vi "VSG25_Main.vi"() -> ()   [LabVIEW 2014]
uses:
  Queue Control.ctl
  sg_lib/VSG25A.lvlib
panel:
  in  "Arb Button":bool
  in  "CW Button":bool
  in  "StepSweep Button":bool
  in  "RampSweep Button":bool
  in  "QAM Button":bool
  in  "FSK Button":bool
  in  "Multitone Button":bool
  in  "Pulse Button":bool
  in  "FM Button":bool
  in  "AM Button":bool
  in  "Exit Button":bool caption="Blank Button"
  in  "Error In":errorcluster
  in  "Connect Button":bool caption="Blank Button"
  out "Error Out":errorcluster
  # "Vector Signal Generator"
  # "Signal Hound VSG25"
  # "Operational Modes:"
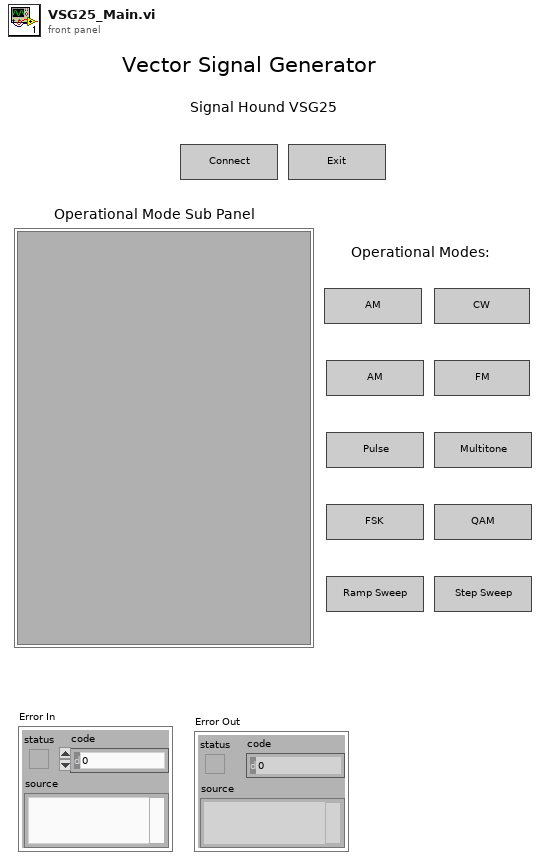
[diagram p1: front panel]
types:
  T1 = typedef "Queue Control.ctl" = cluster{"Command":enum16{"Pulse", "AM", "FM", "Connect", "Exit", "RF On", "CW", "StepSweep", "RampSweep"}, "Data":variant}
  T2 = enum16{"Init", "Proc GUI Events", "Dispatch", "Exit"}
  T3 = enum16{"Pulse", "AM", "FM", "Connect", "Exit", "RF On", "CW", "StepSweep", "RampSweep"}
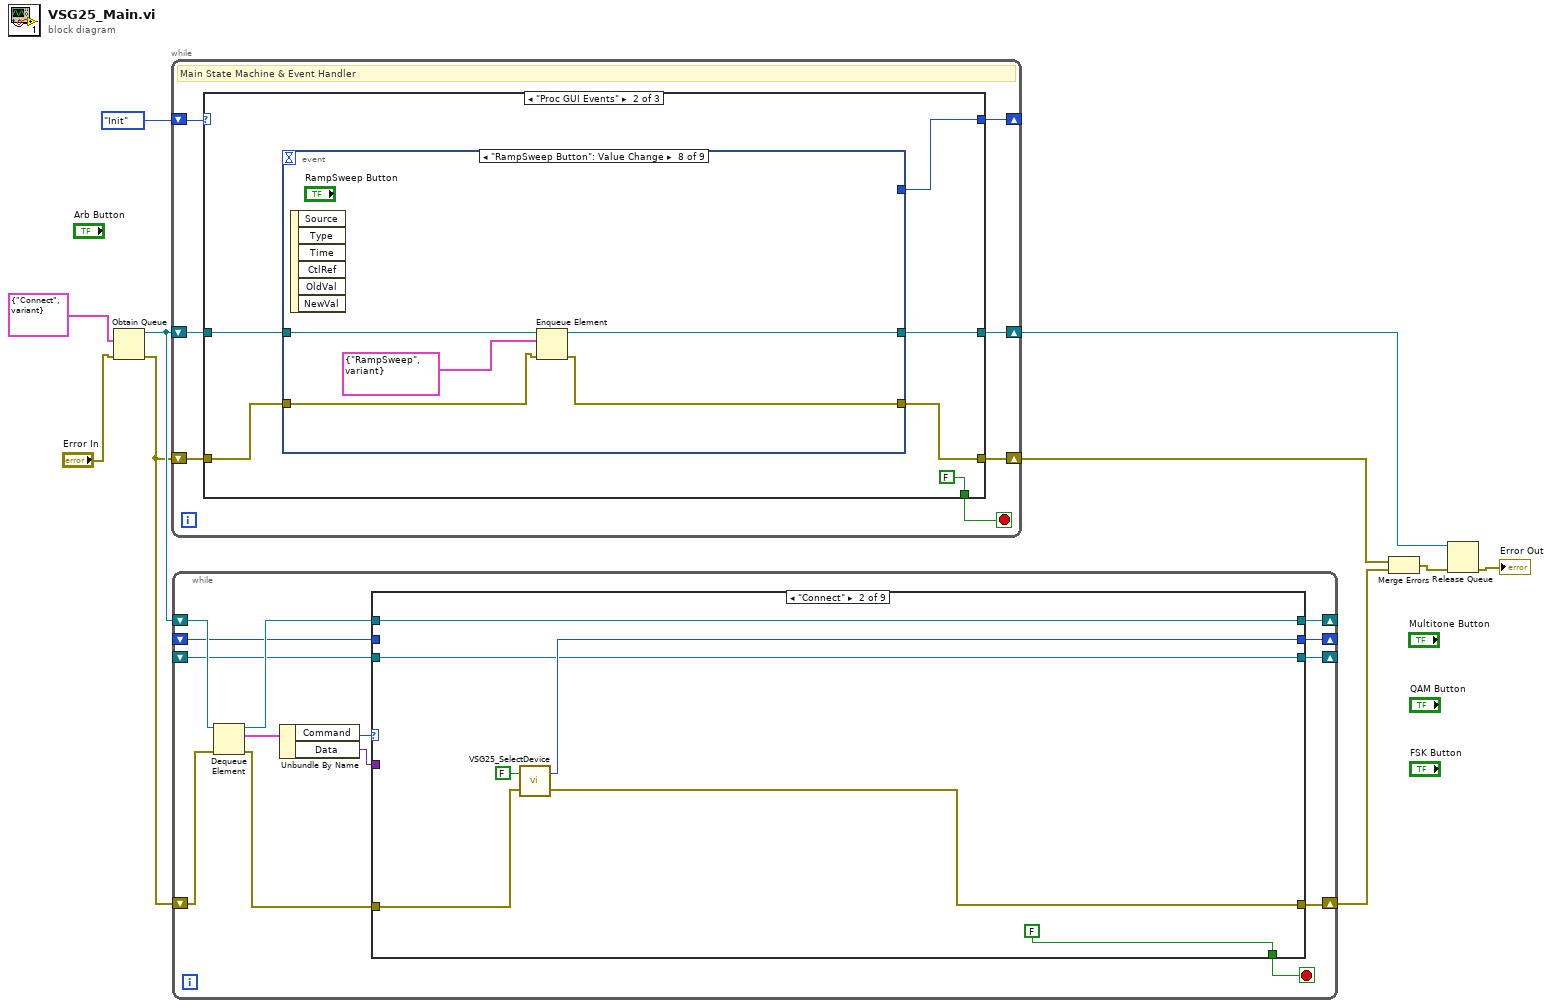
[diagram p0: block diagram]
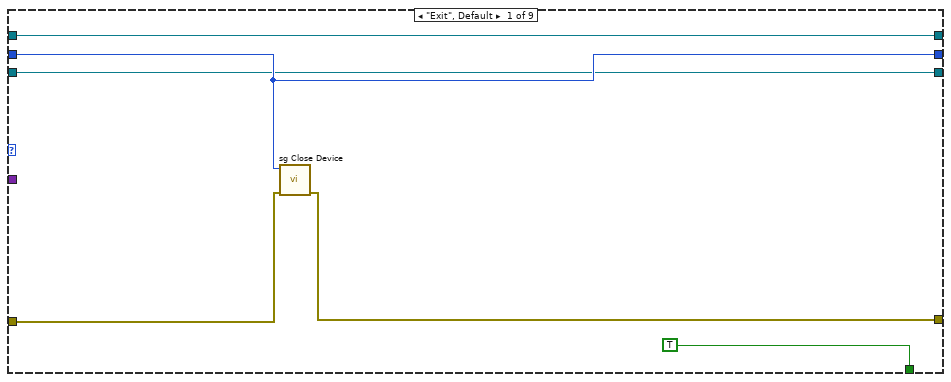
[diagram p2: hidden frame]
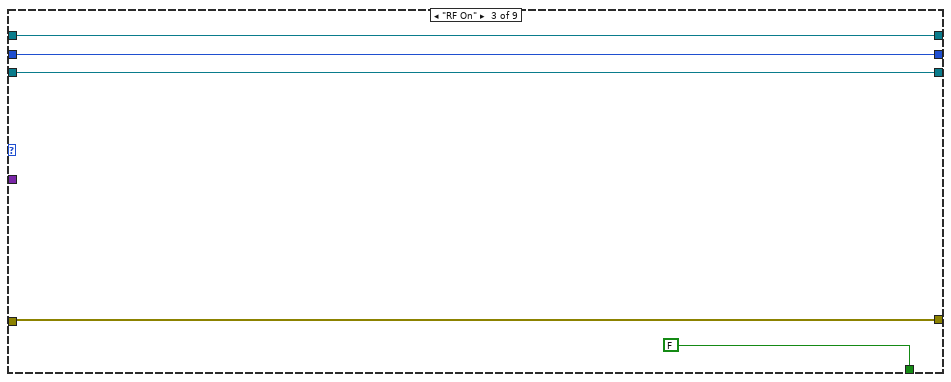
[diagram p3: hidden frame]
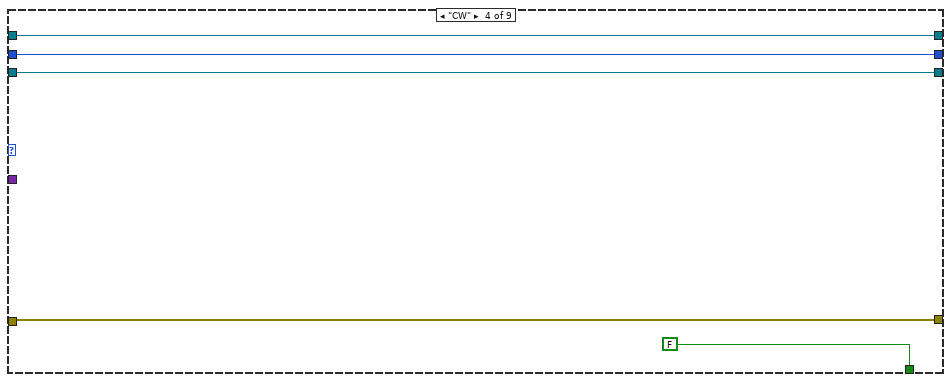
[diagram p4: hidden frame]
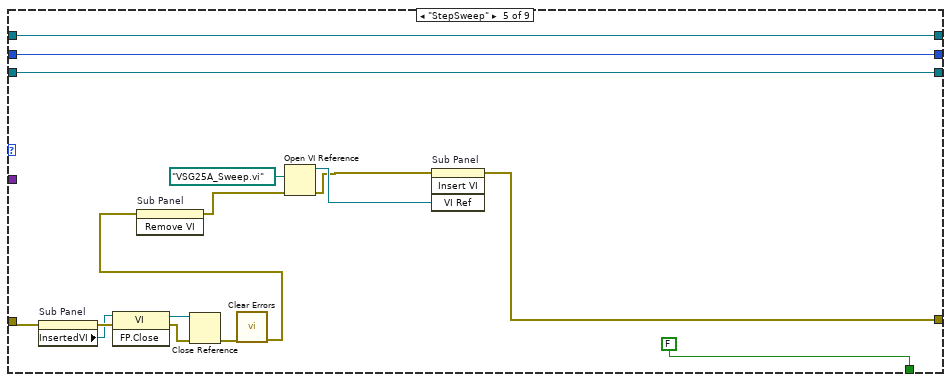
[diagram p5: hidden frame]
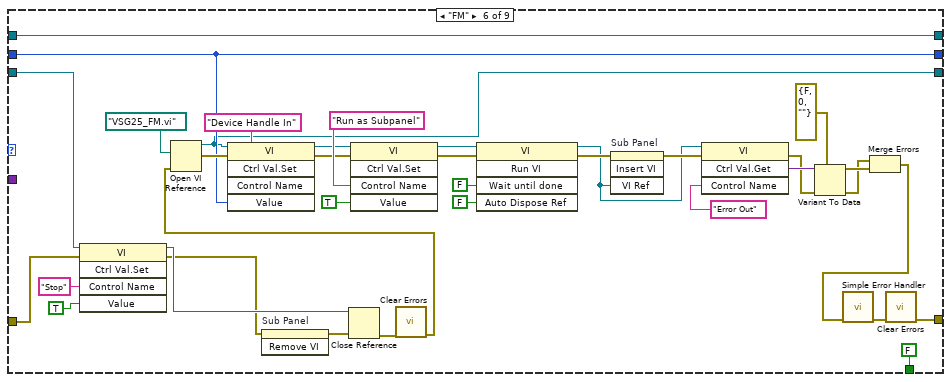
[diagram p6: hidden frame]
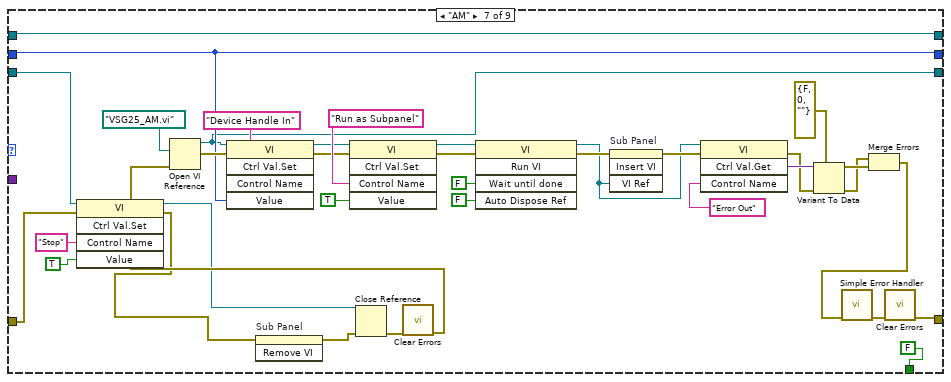
[diagram p7: hidden frame]
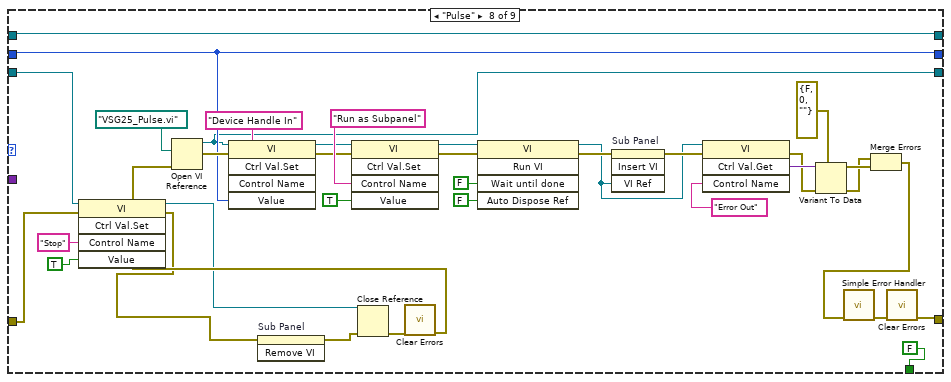
[diagram p8: hidden frame]
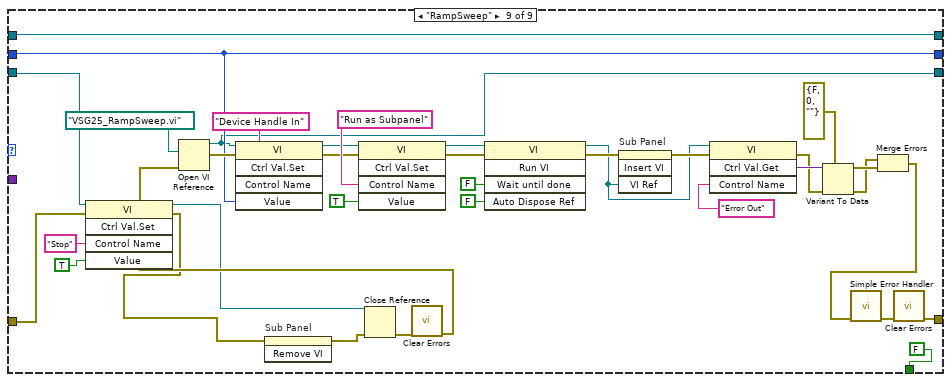
[diagram p9: hidden frame]
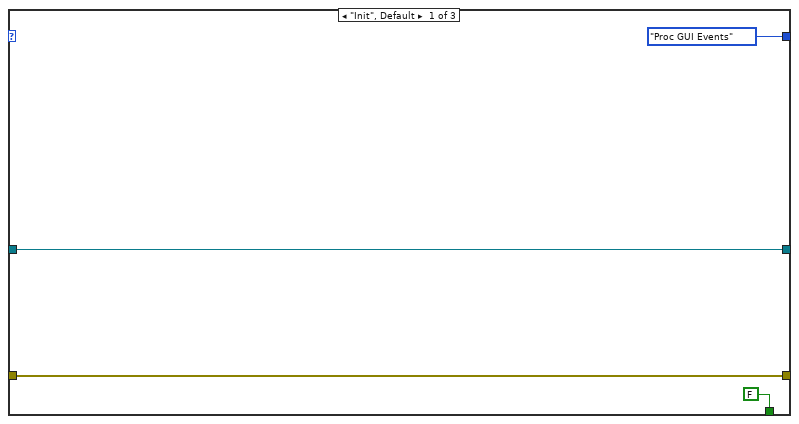
[diagram p10: hidden frame]
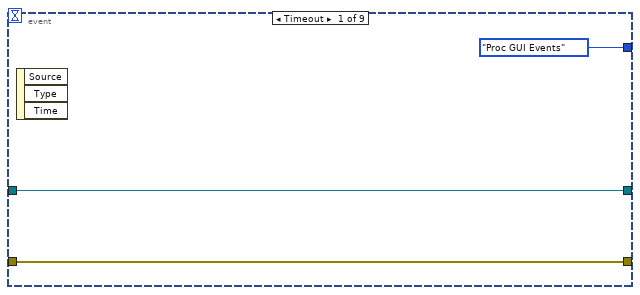
[diagram p11: hidden frame]
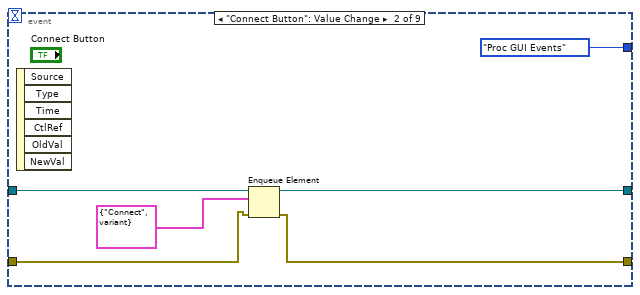
[diagram p12: hidden frame]
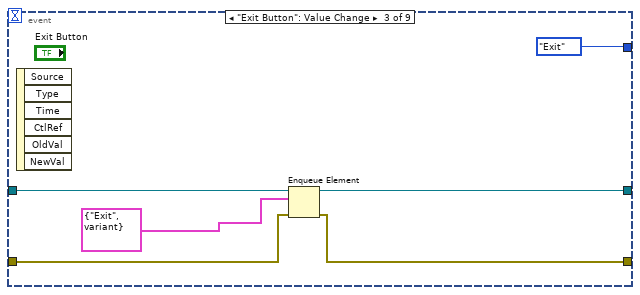
[diagram p13: hidden frame]
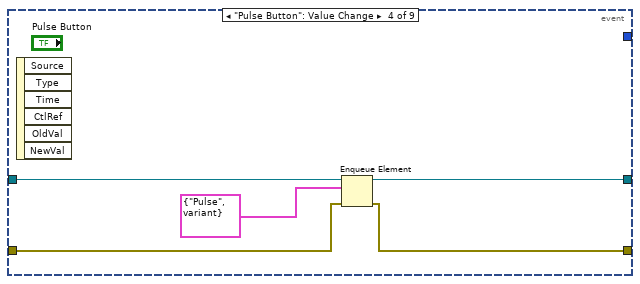
[diagram p14: hidden frame]
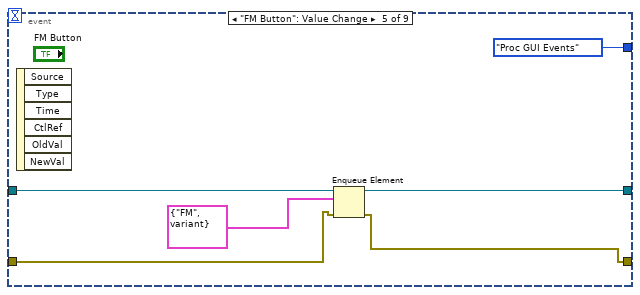
[diagram p15: hidden frame]
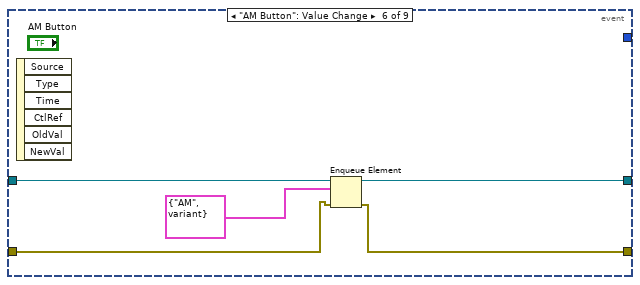
[diagram p16: hidden frame]
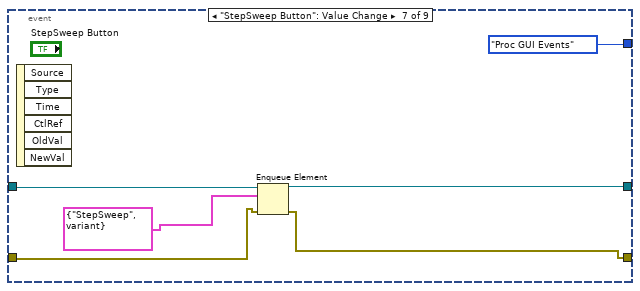
[diagram p17: hidden frame]
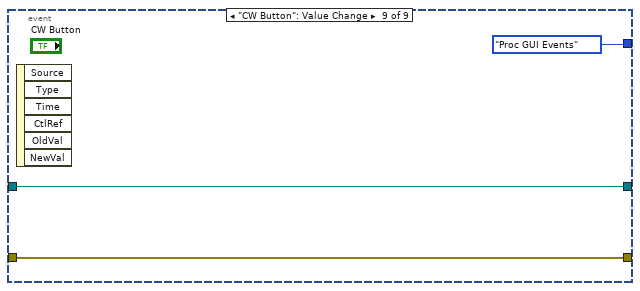
[diagram p18: hidden frame]
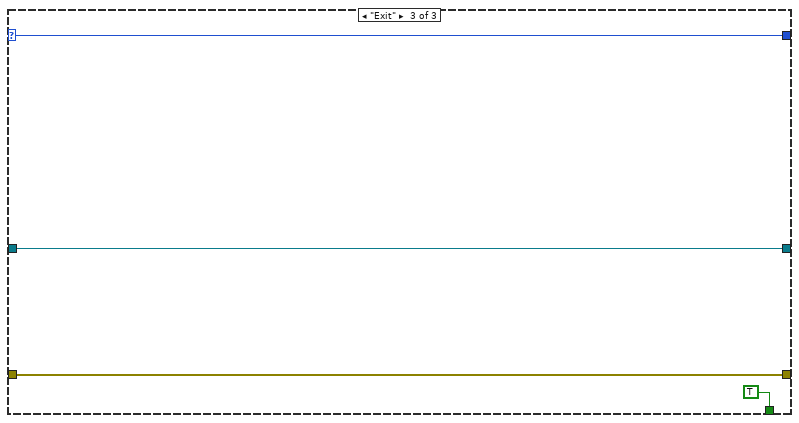
[diagram p19: hidden frame]
diagram:
  n1 = Obtain Queue(element data type=T1 {"Command"=enum."Connect", "Data"=variant} ("Queue Cluster"), error in (no error)="Error In") -> (queue out=w7:refnum<queue>, error out=w1:errorcluster)  [unwired: 3 in, 1 out]
  n2 = while {
    shift-right: [w14] -> _
    shift-left: T2."Init" -> [w17]
    shift-right: [w12] -> w3
    shift-left: w7 -> [w13]
    shift-right: [w11] -> w5
    shift-left: w1 -> [w16]
    stop <- w15 stop-if-true
    # "Main State Machine & Event Handler"
    n3 = case shown="\"Proc GUI Events\"" w17 {
      selector: w17 -> [_ _ w75]
      tunnel: w16 -> [w18 w23 w73]
      tunnel: [FALSE FALSE TRUE] -> w15
      tunnel: [T2."Proc GUI Events" w26 w75] -> w14
      tunnel: w13 -> [w19 w25 w74]
      tunnel: [w19 w24 w74] -> w12
      tunnel: [w18 w22 w73] -> w11
      frame "Init", Default {
      }
      frame "Proc GUI Events" {
        n4 = event shown="[7] \"RampSweep Button\": Value Change" {
          selector: _ -> [_ _ _ _ _ _ _ _ _]
          dyn-events: _ -> [_ _ _ _ _ _ _ _ _]
          timeout: _ -> [_ _ _ _ _ _ _ _ _]
          tunnel: [T2."Proc GUI Events" T2."Proc GUI Events" T2."Exit" _ T2."Proc GUI Events" _ T2."Proc GUI Events" _ T2."Proc GUI Events"] -> w26
          tunnel: w25 -> [w29 w35 w41 w46 w49 w56 w64 w68 w72]
          tunnel: [w29 w34 w40 w43 w50 w57 w61 w65 w72] -> w24
          tunnel: w23 -> [w28 w33 w39 w45 w48 w55 w63 w67 w71]
          tunnel: [w28 w32 w38 w44 w51 w54 w62 w66 w71] -> w22
          event Timeout {
            n5 = event-data() -> ()  [unwired: 1 in, 3 out]
          }
          event "Connect Button": Value Change {
            n6 = event-data() -> ()  [unwired: 1 in, 6 out]
            n7 = Enqueue Element(queue=w35, element=T1 {"Command"=enum."Connect", "Data"=variant} ("Queue Cluster"), error in (no error)=w33) -> (queue out=w34:refnum<queue>, error out=w32:errorcluster)  [unwired: 1 in, 1 out]
          }
          event "Exit Button": Value Change {
            n8 = event-data() -> ()  [unwired: 1 in, 6 out]
            n9 = Enqueue Element(queue=w41, element=T1 {"Command"=enum."Exit", "Data"=variant} ("Queue Cluster"), error in (no error)=w39) -> (queue out=w40:refnum<queue>, error out=w38:errorcluster)  [unwired: 1 in, 1 out]
          }
          event "Pulse Button": Value Change {
            n10 = event-data() -> ()  [unwired: 1 in, 6 out]
            n11 = Enqueue Element(queue=w46, element=T1 {"Command"=enum."Pulse", "Data"=variant} ("Queue Cluster"), error in (no error)=w45) -> (queue out=w43:refnum<queue>, error out=w44:errorcluster)  [unwired: 1 in, 1 out]
          }
          event "FM Button": Value Change {
            n12 = event-data() -> ()  [unwired: 1 in, 6 out]
            n13 = Enqueue Element(queue=w49, element=T1 {"Command"=enum."FM", "Data"=variant} ("Queue Cluster"), error in (no error)=w48) -> (queue out=w50:refnum<queue>, error out=w51:errorcluster)  [unwired: 1 in, 1 out]
          }
          event "AM Button": Value Change {
            n14 = event-data() -> ()  [unwired: 1 in, 6 out]
            n15 = Enqueue Element(queue=w56, element=T1 {"Command"=enum."AM", "Data"=variant} ("Queue Cluster"), error in (no error)=w55) -> (queue out=w57:refnum<queue>, error out=w54:errorcluster)  [unwired: 1 in, 1 out]
          }
          event "StepSweep Button": Value Change {
            n16 = event-data() -> ()  [unwired: 1 in, 6 out]
            n17 = Enqueue Element(queue=w64, element=T1 {"Command"=enum."StepSweep", "Data"=variant} ("Queue Cluster"), error in (no error)=w63) -> (queue out=w61:refnum<queue>, error out=w62:errorcluster)  [unwired: 1 in, 1 out]
          }
          event "RampSweep Button": Value Change {
            n18 = event-data() -> ()  [unwired: 1 in, 6 out]
            n19 = Enqueue Element(queue=w68, element=T1 {"Command"=enum."RampSweep", "Data"=variant} ("Queue Cluster"), error in (no error)=w67) -> (queue out=w65:refnum<queue>, error out=w66:errorcluster)  [unwired: 1 in, 1 out]
          }
          event "CW Button": Value Change {
            n20 = event-data() -> ()  [unwired: 1 in, 6 out]
          }
        }
      }
      frame "Exit" {
      }
    }
  }
  n21 = while {
    shift-right: [w88] -> _
    shift-left: w7 -> [w90]
    shift-right: [w86] -> w6
    shift-left: w1 -> [w85]
    shift-right: [w82] -> _
    shift-left: _ -> [w81]
    shift-right: [w78] -> _
    shift-left: _ -> [w77]
    stop <- w80 stop-if-true
    n22 = Dequeue Element(queue=w90, error in (no error)=w85) -> (queue out=w89:refnum<queue>, element=w84:T1, error out=w87:errorcluster)  [unwired: 1 in, 1 out]
    n23 = Unbundle By Name(w84) -> ("Command"=w83:T3, "Data"=w79:variant)
    n24 = case shown="\"Connect\"" w83 {
      tunnel: w89 -> [w93 w103 w106 w111 w124 w164 w177 w205 w243]
      tunnel: [w93 w103 w106 w111 w124 w164 w177 w205 w243] -> w88
      tunnel: w87 -> [w95 w102 w105 w110 w116 w130 w166 w207 w240]
      tunnel: [w94 w98 w105 w110 w122 w139 w175 w202 w239] -> w86
      tunnel: [w96 w101 w107 w112 w125 w156 w178 w204 w242] -> w82
      tunnel: w81 -> [w96 _ w107 w112 w125 w156 w178 w204 w242]
      tunnel: [TRUE ("AutoSel") FALSE ("AutoSel") FALSE ("AutoSel") FALSE ("AutoSel") FALSE ("AutoSel") FALSE ("AutoSel") FALSE ("AutoSel") FALSE ("AutoSel") FALSE ("AutoSel")] -> w80
      tunnel: w79 -> [_ _ _ _ _ _ _ _ _]
      tunnel: [w91 w97 w104 w109 w114 w137 w173 w203 w241] -> w78
      tunnel: w77 -> [w91 w97 w104 w109 w114 w131 w170 w206 w244]
      frame "Exit", Default {
        n25 = call "sg Close Device.vi"("error in (no error)"=w95, "device"=w96) -> ("error out"=w94:errorcluster)  [unwired: 8 in, 1 out]
      }
      frame "Connect" {
        n26 = call "VSG25_SelectDevice.vi"("ErrorIn"=w102, "AutoSel"=FALSE) -> ("ErrorOut"=w98:errorcluster, "deviceHandle"=w101:i32)
      }
      frame "RF On" {
      }
      frame "CW" {
      }
      frame "StepSweep" {
        n27 = property on="Sub Panel" class="SubPnl"(error in=w116) -> (error out=w119:errorcluster, "InsertedVI"=w118:refnum<vi>)  [unwired: 1 in, 1 out]
        n28 = invoke class="VI" method="FP.Close"(reference=w118, error in=w119) -> (reference out=w121:refnum<vi>, error out=w120:errorcluster)  [unwired: 1 in, 1 out]
        n29 = Close Reference(reference=w121, error in (no error)=w120) -> (error out=w117:errorcluster)
        n30 = call <vilib>:"Clear Errors.vi"("error in (no error)"=w117) -> ("error out"=w115:errorcluster)  [unwired: 5 in, 1 out]
        n31 = invoke on="Sub Panel" class="SubPnl" method="Remove VI"(error in=w115) -> (error out=w123:errorcluster)  [unwired: 2 in, 2 out]
        n32 = Open VI Reference(vi path=path "VSG25A_Sweep.vi", error in (no error)=w123) -> (vi reference=w128:refnum<vi>, error out=w127:errorcluster)  [unwired: 4 in]
        n33 = invoke on="Sub Panel" class="SubPanel" method="Insert VI"(error in=w127, "VI Ref"=w128) -> (error out=w122:errorcluster)  [unwired: 2 in, 3 out]
      }
      frame "FM" {
        n34 = invoke class="VI" method="Ctrl Val.Set"(reference=w131, error in=w130, "Control Name"="Stop", "Value"=TRUE) -> (reference out=w133:refnum<vi>, error out=w132:errorcluster)  [unwired: 1 in, 3 out]
        n35 = invoke on="Sub Panel" class="SubPnl" method="Remove VI"(error in=w132) -> (error out=w136:errorcluster)  [unwired: 2 in, 2 out]
        n36 = Close Reference(reference=w133, error in (no error)=w136) -> (error out=w142:errorcluster)
        n37 = call <vilib>:"Clear Errors.vi"("error in (no error)"=w142) -> ("error out"=w138:errorcluster)  [unwired: 5 in, 1 out]
        n38 = Open VI Reference(vi path=path "VSG25_FM.vi", error in (no error)=w138) -> (vi reference=w137:refnum<vi>, error out=w159:errorcluster)  [unwired: 4 in]
        n39 = invoke class="VI" method="Ctrl Val.Set"(reference=w137, error in=w159, "Control Name"="Device Handle In", "Value"=w156) -> (reference out=w157:refnum<vi>, error out=w158:errorcluster)  [unwired: 1 in, 3 out]
        n40 = invoke class="VI" method="Ctrl Val.Set"(reference=w157, error in=w158, "Control Name"="Run as Subpanel", "Value"=TRUE) -> (reference out=w155:refnum<vi>, error out=w152:errorcluster)  [unwired: 1 in, 3 out]
        n41 = invoke class="VI" method="Run VI"(reference=w155, error in=w152, "Wait until done"=FALSE ("Wait Until Done"), "Auto Dispose Ref"=FALSE ("Auto Dispose Reference")) -> (reference out=w148:refnum<vi>, error out=w151:errorcluster)  [unwired: 1 in, 3 out]
        n42 = invoke on="Sub Panel" class="SubPanel" method="Insert VI"(error in=w151, "VI Ref"=w148) -> (error out=w149:errorcluster)  [unwired: 2 in, 3 out]
        n43 = invoke class="VI" method="Ctrl Val.Get"(reference=w148, error in=w149, "Control Name"="Error Out") -> (error out=w144:errorcluster, "Get Control Value Variant"=w147:variant)  [unwired: 1 in, 2 out]
        n44 = Variant To Data(error in=w144, type=errorcluster {"status"=FALSE, "code"=0, "source"=""} ("error constant"), Variant=w147) -> (data=w145:errorcluster, error out=w143:errorcluster)
        n45 = Merge Errors(w143, w145) -> (w141:errorcluster)
        n46 = call <vilib>:"Simple Error Handler.vi"("error in (no error)"=w141) -> ("error out"=w140:errorcluster)  [unwired: 4 in, 4 out]
        n47 = call <vilib>:"Clear Errors.vi"("error in (no error)"=w140) -> ("error out"=w139:errorcluster)  [unwired: 5 in, 1 out]
      }
      frame "AM" {
        n48 = invoke class="VI" method="Ctrl Val.Set"(reference=w170, error in=w166, "Control Name"="Stop", "Value"=TRUE) -> (reference out=w168:refnum<vi>, error out=w167:errorcluster)  [unwired: 1 in, 3 out]
        n49 = invoke on="Sub Panel" class="SubPnl" method="Remove VI"(error in=w167) -> (error out=w169:errorcluster)  [unwired: 2 in, 2 out]
        n50 = Close Reference(reference=w168, error in (no error)=w169) -> (error out=w181:errorcluster)
        n51 = call <vilib>:"Clear Errors.vi"("error in (no error)"=w181) -> ("error out"=w174:errorcluster)  [unwired: 5 in, 1 out]
        n52 = Open VI Reference(vi path=path "VSG25_AM.vi", error in (no error)=w174) -> (vi reference=w173:refnum<vi>, error out=w197:errorcluster)  [unwired: 4 in]
        n53 = invoke class="VI" method="Ctrl Val.Set"(reference=w173, error in=w197, "Control Name"="Device Handle In", "Value"=w178) -> (reference out=w195:refnum<vi>, error out=w196:errorcluster)  [unwired: 1 in, 3 out]
        n54 = invoke class="VI" method="Ctrl Val.Set"(reference=w195, error in=w196, "Control Name"="Run as Subpanel", "Value"=TRUE) -> (reference out=w194:refnum<vi>, error out=w191:errorcluster)  [unwired: 1 in, 3 out]
        n55 = invoke class="VI" method="Run VI"(reference=w194, error in=w191, "Wait until done"=FALSE ("Wait Until Done"), "Auto Dispose Ref"=FALSE ("Auto Dispose Reference")) -> (reference out=w187:refnum<vi>, error out=w190:errorcluster)  [unwired: 1 in, 3 out]
        n56 = invoke on="Sub Panel" class="SubPanel" method="Insert VI"(error in=w190, "VI Ref"=w187) -> (error out=w188:errorcluster)  [unwired: 2 in, 3 out]
        n57 = invoke class="VI" method="Ctrl Val.Get"(reference=w187, error in=w188, "Control Name"="Error Out") -> (error out=w183:errorcluster, "Get Control Value Variant"=w186:variant)  [unwired: 1 in, 2 out]
        n58 = Variant To Data(error in=w183, type=errorcluster {"status"=FALSE, "code"=0, "source"=""} ("error constant"), Variant=w186) -> (data=w184:errorcluster, error out=w182:errorcluster)
        n59 = Merge Errors(w182, w184) -> (w180:errorcluster)
        n60 = call <vilib>:"Simple Error Handler.vi"("error in (no error)"=w180) -> ("error out"=w179:errorcluster)  [unwired: 4 in, 4 out]
        n61 = call <vilib>:"Clear Errors.vi"("error in (no error)"=w179) -> ("error out"=w175:errorcluster)  [unwired: 5 in, 1 out]
      }
      frame "Pulse" {
        n62 = invoke class="VI" method="Ctrl Val.Set"(reference=w206, error in=w207, "Control Name"="Stop", "Value"=TRUE) -> (reference out=w210:refnum<vi>, error out=w209:errorcluster)  [unwired: 1 in, 3 out]
        n63 = invoke on="Sub Panel" class="SubPnl" method="Remove VI"(error in=w209) -> (error out=w211:errorcluster)  [unwired: 2 in, 2 out]
        n64 = Close Reference(reference=w210, error in (no error)=w211) -> (error out=w217:errorcluster)
        n65 = call <vilib>:"Clear Errors.vi"("error in (no error)"=w217) -> ("error out"=w214:errorcluster)  [unwired: 5 in, 1 out]
        n66 = Open VI Reference(vi path=path "VSG25_Pulse.vi", error in (no error)=w214) -> (vi reference=w203:refnum<vi>, error out=w233:errorcluster)  [unwired: 4 in]
        n67 = invoke class="VI" method="Ctrl Val.Set"(reference=w203, error in=w233, "Control Name"="Device Handle In", "Value"=w204) -> (reference out=w231:refnum<vi>, error out=w232:errorcluster)  [unwired: 1 in, 3 out]
        n68 = invoke class="VI" method="Ctrl Val.Set"(reference=w231, error in=w232, "Control Name"="Run as Subpanel", "Value"=TRUE) -> (reference out=w230:refnum<vi>, error out=w227:errorcluster)  [unwired: 1 in, 3 out]
        n69 = invoke class="VI" method="Run VI"(reference=w230, error in=w227, "Wait until done"=FALSE ("Wait Until Done"), "Auto Dispose Ref"=FALSE ("Auto Dispose Reference")) -> (reference out=w223:refnum<vi>, error out=w226:errorcluster)  [unwired: 1 in, 3 out]
        n70 = invoke on="Sub Panel" class="SubPanel" method="Insert VI"(error in=w226, "VI Ref"=w223) -> (error out=w224:errorcluster)  [unwired: 2 in, 3 out]
        n71 = invoke class="VI" method="Ctrl Val.Get"(reference=w223, error in=w224, "Control Name"="Error Out") -> (error out=w219:errorcluster, "Get Control Value Variant"=w222:variant)  [unwired: 1 in, 2 out]
        n72 = Variant To Data(error in=w219, type=errorcluster {"status"=FALSE, "code"=0, "source"=""} ("error constant"), Variant=w222) -> (data=w220:errorcluster, error out=w218:errorcluster)
        n73 = Merge Errors(w218, w220) -> (w216:errorcluster)
        n74 = call <vilib>:"Simple Error Handler.vi"("error in (no error)"=w216) -> ("error out"=w215:errorcluster)  [unwired: 4 in, 4 out]
        n75 = call <vilib>:"Clear Errors.vi"("error in (no error)"=w215) -> ("error out"=w202:errorcluster)  [unwired: 5 in, 1 out]
      }
      frame "RampSweep" {
        n76 = invoke class="VI" method="Ctrl Val.Set"(reference=w244, error in=w240, "Control Name"="Stop", "Value"=TRUE) -> (reference out=w246:refnum<vi>, error out=w245:errorcluster)  [unwired: 1 in, 3 out]
        n77 = invoke on="Sub Panel" class="SubPnl" method="Remove VI"(error in=w245) -> (error out=w247:errorcluster)  [unwired: 2 in, 2 out]
        n78 = Close Reference(reference=w246, error in (no error)=w247) -> (error out=w253:errorcluster)
        n79 = call <vilib>:"Clear Errors.vi"("error in (no error)"=w253) -> ("error out"=w250:errorcluster)  [unwired: 5 in, 1 out]
        n80 = Open VI Reference(vi path=path "VSG25_RampSweep.vi", error in (no error)=w250) -> (vi reference=w241:refnum<vi>, error out=w269:errorcluster)  [unwired: 4 in]
        n81 = invoke class="VI" method="Ctrl Val.Set"(reference=w241, error in=w269, "Control Name"="Device Handle In", "Value"=w242) -> (reference out=w267:refnum<vi>, error out=w268:errorcluster)  [unwired: 1 in, 3 out]
        n82 = invoke class="VI" method="Ctrl Val.Set"(reference=w267, error in=w268, "Control Name"="Run as Subpanel", "Value"=TRUE) -> (reference out=w266:refnum<vi>, error out=w263:errorcluster)  [unwired: 1 in, 3 out]
        n83 = invoke class="VI" method="Run VI"(reference=w266, error in=w263, "Wait until done"=FALSE ("Wait Until Done"), "Auto Dispose Ref"=FALSE ("Auto Dispose Reference")) -> (reference out=w259:refnum<vi>, error out=w262:errorcluster)  [unwired: 1 in, 3 out]
        n84 = invoke on="Sub Panel" class="SubPanel" method="Insert VI"(error in=w262, "VI Ref"=w259) -> (error out=w260:errorcluster)  [unwired: 2 in, 3 out]
        n85 = invoke class="VI" method="Ctrl Val.Get"(reference=w259, error in=w260, "Control Name"="Error Out") -> (error out=w255:errorcluster, "Get Control Value Variant"=w258:variant)  [unwired: 1 in, 2 out]
        n86 = Variant To Data(error in=w255, type=errorcluster {"status"=FALSE, "code"=0, "source"=""} ("error constant"), Variant=w258) -> (data=w256:errorcluster, error out=w254:errorcluster)
        n87 = Merge Errors(w254, w256) -> (w252:errorcluster)
        n88 = call <vilib>:"Simple Error Handler.vi"("error in (no error)"=w252) -> ("error out"=w251:errorcluster)  [unwired: 4 in, 4 out]
        n89 = call <vilib>:"Clear Errors.vi"("error in (no error)"=w251) -> ("error out"=w239:errorcluster)  [unwired: 5 in, 1 out]
      }
    }
  }
  n90 = Merge Errors(w5, w6) -> (w4:errorcluster)
  n91 = Release Queue(queue=w3, error in (no error)=w4) -> (error out=→"Error Out":errorcluster)  [unwired: 1 in, 2 out]
